vi "SetActualPosition.vi"(8 "error in (no error)":errorcluster) -> (0 "error out":errorcluster)   [LabVIEW 2020, in "输出轴伺服.lvlib"]
uses:
  Servo_global.vi
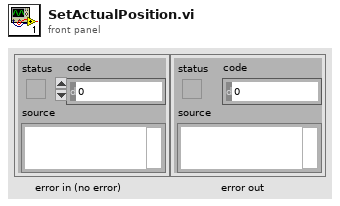
[diagram p1: front panel]
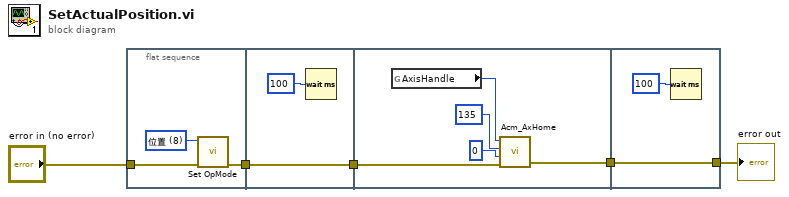
[diagram p0: block diagram]
diagram:
  n1 = flat-sequence {
    tunnel: "error in (no error)" -> [w7]
    tunnel: [w6] -> w4
    tunnel: w4 -> [w10]
    tunnel: [w10] -> w3
    tunnel: w3 -> [w14]
    tunnel: [w11] -> w1
    tunnel: [w17] -> w2
    tunnel: w1 -> [w17]
    frame #0 {
      w8 = u32 8 items=["位置"=8, "速度"=9, "扭矩"=10] ("Value")
      n2 = call "Set OpMode.vi"("error in (no error)"=w7, "Value"=w8) -> ("error out"=w6:errorcluster)  [unwired: 9 in]
    }
    frame #1 {
      n3 = Wait (ms)(milliseconds to wait=u32 100 ("等待时间（毫秒）")) -> ()  [unwired: 1 out]
    }
    frame #2 {
      n4 = global read "Servo_global.vi" "AxisHandle"() -> (w15:u32)
      n5 = call <userlib>:"Acm_AxHome.vi"("error in (no error)"=w14, "DirMode"=u32 0, "HomeMode"=u32 135, "AxisHandle"=w15) -> ("error out"=w11:errorcluster)  [unwired: 2 out]
    }
    frame #3 {
      n6 = Wait (ms)(milliseconds to wait=u32 100 ("等待时间（毫秒）")) -> ()  [unwired: 1 out]
    }
  }
  "error out" <- w2
